vi "PromptUserWithDefault.vi"(7 "is Category?":bool, 9 "Recommended Name (\"\": None)":string, 10 "Structure Type":T1, 11 "Section":string) -> (1 "OK":bool, 2 "NewTag 2":string caption="NewTag")   [LabVIEW 2013]
uses:
  StructureTypes.ctl
panel:
  in  "New Frame Name":string caption="NewTag"
  out "error out":errorcluster
  in  "error in (no error)":errorcluster
  out "String":string="Enter new case name or hit 'Cancel'."
  in  "Enable":bool=TRUE
  in  "Cancel":bool
  in  "OK2":bool
  in  "OK1":bool
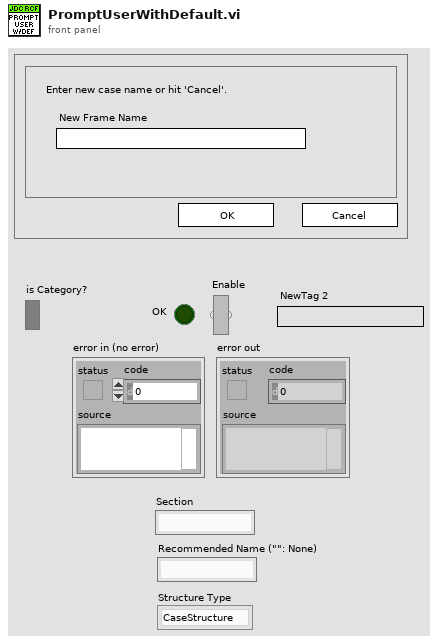
[diagram p1: front panel]
types:
  T1 = typedef "StructureTypes.ctl" = enum16{"CaseStructure", "EventStructure"}
  T2 = cluster{"Selection Start":u32, "Selection End":u32}
  T3 = cluster{"Input Name":string, "Input Data Type":i32}[]
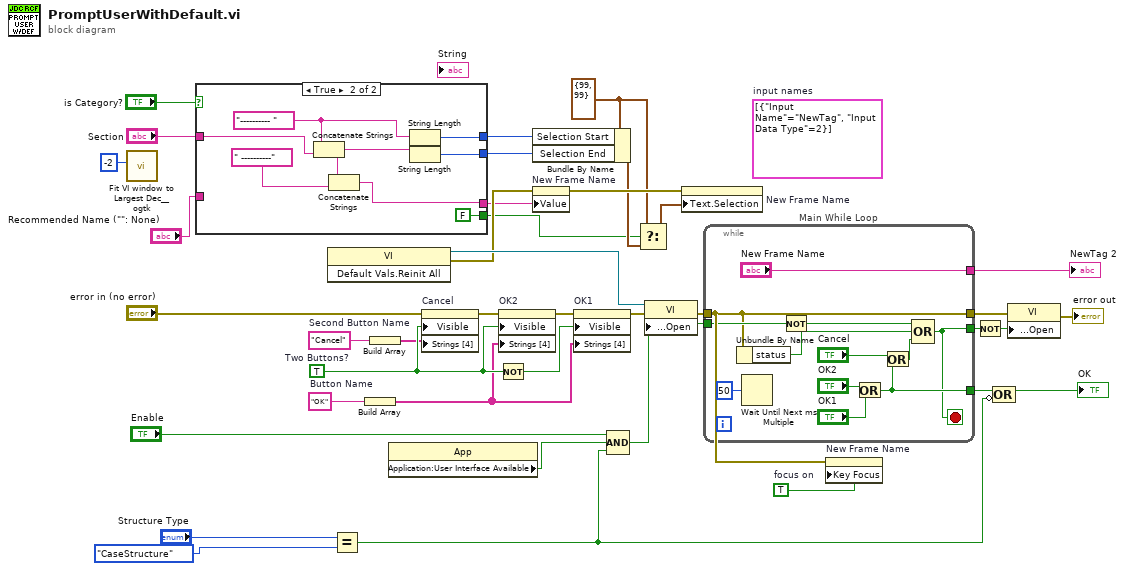
[diagram p0: block diagram]
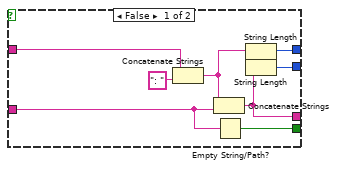
[diagram p2: hidden frame]
diagram:
  w6 = T2 {"Selection Start"=99, "Selection End"=99} ("Text.Selection")
  w23 = TRUE  # focus on
  (unwired) T3 [{"Input Name"="NewTag", "Input Data Type"=2}]  # input names
  w32 = "Cancel"  # Second Button Name
  w30 = "OK"  # Button Name
  w39 = TRUE  # Two Buttons?
  n1 = call <userlib>:"Fit VI window to Largest Dec__ogtk.vi"("border spacing (2 px)"=-2) -> ()  [unwired: 5 in, 2 out]
  n2 = case shown="True" "is Category?" {
    tunnel: "Section" -> [w46 w53]
    tunnel: "Recommended Name (\"\": None)" -> [w41 _]
    tunnel: [w44 w48] -> w7
    tunnel: [w43 w51] -> w4
    tunnel: [w42 w55] -> w3
    tunnel: [w40 FALSE] -> w1
    frame False {
      n3 = Concatenate Strings(w46, ": " ("string")) -> (w45:string)
      n4 = Concatenate Strings(w45, w41) -> (w44:string)
      n5 = Empty String/Path?(string/path=w41) -> (empty?=w40:bool)
      n6 = String Length(string=w45) -> (length=w43:i32)
      n7 = String Length(string=w44) -> (length=w42:i32)
    }
    frame True {
      w50 = "---------- " ("Section")
      n8 = Concatenate Strings(w50, w53) -> (w49:string)
      n9 = Concatenate Strings(w49, " ----------" ("Section")) -> (w48:string)
      n10 = String Length(string=w50) -> (length=w51:i32)
      n11 = String Length(string=w49) -> (length=w55:i32)
    }
  }
  n12 = invoke class="VI" method="Default Vals.Reinit All"() -> (reference out=w24:refnum<vi>, error out=w16:errorcluster)  [unwired: 3 in, 1 out]
  n13 = Equal?(x="Structure Type", y=StructureTypes."CaseStructure") -> (x = y?=w11:bool)
  n14 = Build Array(w30) -> (w31:string[])
  n15 = Build Array(w32) -> (w33:string[])
  n16 = property class="App"() -> ("Application:User Interface Available"=w25:bool)  [unwired: 2 in, 2 out]
  n17 = property on="Cancel" class="Bool"(error in="error in (no error)", "Visible"=w39, "Strings [4]"=w33) -> (error out=w37:errorcluster)  [unwired: 1 in, 1 out]
  n18 = Not(x=w39) -> (.not. x?=w38:bool)
  n19 = property on="OK2" class="Bool"(error in=w37, "Visible"=w39, "Strings [4]"=w31) -> (error out=w36:errorcluster)  [unwired: 1 in, 1 out]
  n20 = Bundle By Name(cluster=w6, "Selection Start"=w4, "Selection End"=w3) -> (w5:T2)
  n21 = property on="New Frame Name" class="Str"(error in=w16, "Value"=w7) -> (error out=w15:errorcluster)  [unwired: 1 in, 1 out]
  n22 = property on="OK1" class="Bool"(error in=w36, "Visible"=w38, "Strings [4]"=w31) -> (error out=w29:errorcluster)  [unwired: 1 in, 1 out]
  n23 = Compound Arithmetic op=AND("Enable", w25, w11) -> (w26:bool)
  n24 = Select(t=w6, s=w1, f=w5) -> (s? t:f=w8:T2)
  n25 = property class="VI"(reference=w24, error in=w29, "Front Panel Window:Open"=w26) -> (error out=w28:errorcluster)  [unwired: 1 out]
  n26 = property on="New Frame Name" class="Str"(error in=w15, "Text.Selection"=w8) -> ()  [unwired: 1 in, 2 out]
  n27 = while "Main While Loop" {
    tunnel: [w66] -> w20
    tunnel: w26 -> [w65]
    tunnel: [w63] -> w34
    tunnel: w28 -> [w62]
    tunnel: [w62] -> w27
    tunnel: ["New Frame Name"] -> w18
    stop <- w63 stop-if-true
    n28 = Unbundle By Name(w62) -> ("status"=w60:bool)
    n29 = Wait Until Next ms Multiple(millisecond multiple=u32 50) -> ()  [unwired: 1 out]
    n30 = Not(x=w65) -> (.not. x?=w64:bool)
    n31 = Or(x="OK2", y="OK1") -> (x .or. y?=w66:bool)
    n32 = Or(x="Cancel", y=w66) -> (x .or. y?=w61:bool)
    n33 = Compound Arithmetic op=OR(w64, w60, w61) -> (w63:bool)
  }
  "NewTag 2" <- w18
  n34 = property on="New Frame Name" class="Str"(error in=w28, "Key Focus"=w23) -> ()  [unwired: 1 in, 2 out]
  n35 = Not(x=w34) -> (.not. x?=w35:bool)
  n36 = Compound Arithmetic op=OR(w20, invert w11) -> (→"OK":bool)
  n37 = property class="VI"(error in=w27, "Front Panel Window:Open"=w35) -> (error out=→"error out":errorcluster)  [unwired: 1 in, 1 out]
